vi "0037-0001_SHT31.vi"() -> ()   [LabVIEW 2014]
panel:
  out "x = y?":bool
  out "湿度":dbl format="%.2g"
  out "温度":dbl format="%.2g"
  in  "停止ボタン":bool
  # "℃"
  # "％RH"
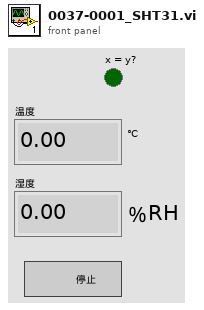
[diagram p1: front panel]
types:
  T1 = cluster{"bitRate":u32, "address":u8, "autoReadRespond":bool, "writeTimeout":u16, "readTimeout":u16, "sclLowTimeout":bool, "transferRetries":u16}
  T2 = typedef "CP2112_device.ctl" = i32
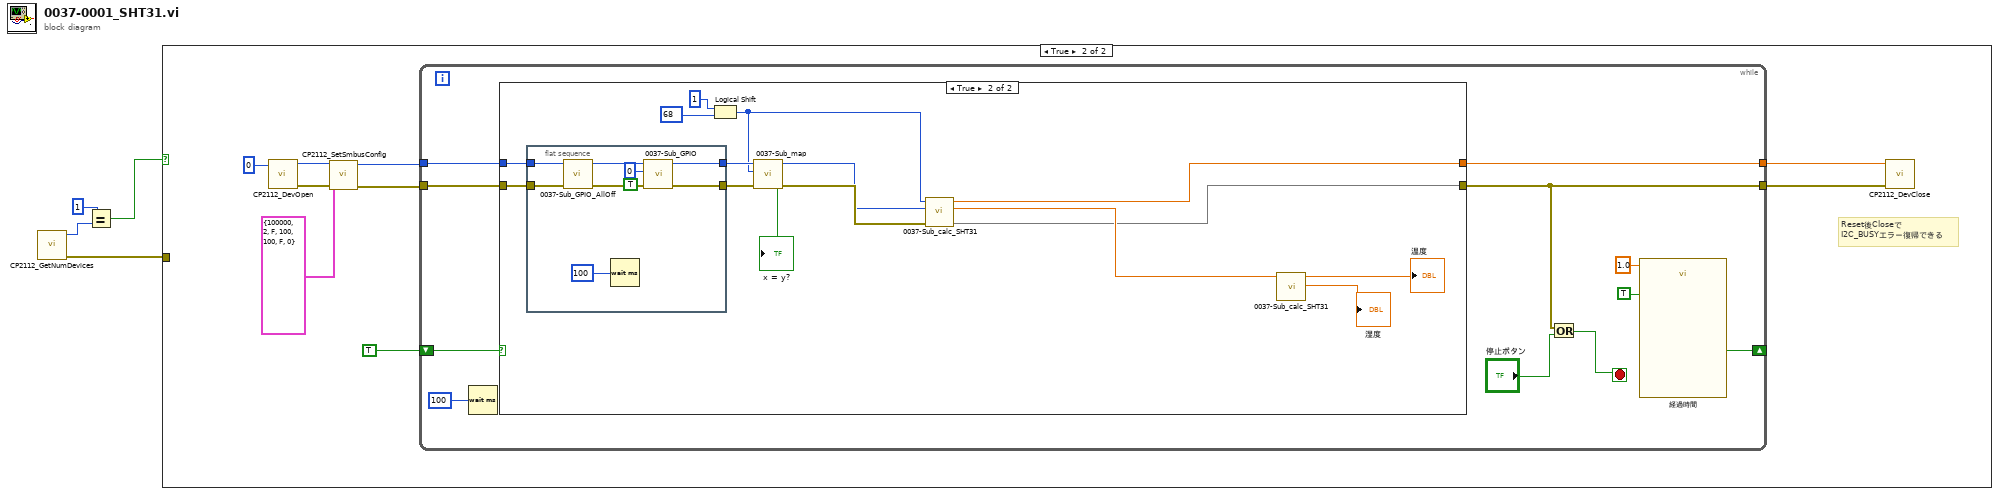
[diagram p0: block diagram]
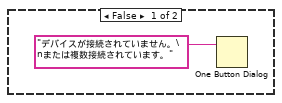
[diagram p2: hidden frame]
diagram:
  n1 = call <userlib>:"CP2112_GetNumDevices.vi"() -> ("error out"=w1:errorcluster, "numDevices"=w3:i32)  [unwired: 9 in, 1 out]
  n2 = Equal?(x=1, y=w3) -> (x = y?=w2:bool)
  n3 = case shown="TRUE" w2 {
    tunnel: w1 -> [_ _]
    frame False {
      n4 = One Button Dialog(message="デバイスが接続されていません。\nまたは複数接続されています。" ("メッセージ")) -> ()  [unwired: 1 in, 1 out]
    }
    frame True {
      # "Reset後Closeで\nI2C_BUSYエラー復帰できる"
      n5 = call <userlib>:"CP2112_DevOpen.vi"("deviceNum"=0) -> ("error out"=w9:errorcluster, "device"=w10:T2)  [unwired: 8 in, 1 out]
      n6 = call <userlib>:"CP2112_SetSmbusConfig.vi"("error in (no error)"=w9, "smbusInfo"=T1 {"bitRate"=100000, "address"=2, "autoReadRespond"=FALSE, "writeTimeout"=100, "readTimeout"=100, "sclLowTimeout"=FALSE, "transferRetries"=0}, "device"=w10) -> ("error out"=w11:errorcluster, "deviceOut"=w12:T2)  [unwired: 6 in, 1 out]
      n7 = while {
        tunnel: w11 -> [w25]
        tunnel: w12 -> [w24]
        tunnel: [w21] -> w7
        tunnel: [w20] -> w6
        shift-right: [w17] -> _
        shift-left: TRUE ("Auto Reset") -> [w18]
        stop <- w22 stop-if-true
        n8 = Wait (ms)(milliseconds to wait=u32 100 ("ミリ秒待機時間")) -> ()  [unwired: 1 out]
        n9 = case shown="TRUE" w18 {
          tunnel: w25 -> [w26 w33]
          tunnel: w24 -> [w27 w34]
          tunnel: [w26 w36] -> w21
          tunnel: [w27 w35] -> w20
          frame False {
          }
          frame True {
            n10 = flat-sequence {
              tunnel: w34 -> [w51]
              tunnel: w33 -> [w48]
              tunnel: [w49] -> w32
              tunnel: [w46] -> w31
              frame #0 {
                n11 = call "0037-Sub_GPIO_AllOff.vi"("エラー出力 2"=w48, "device"=w51) -> ("エラー出力"=w47:errorcluster, "deviceOut"=w50:T2)  [unwired: 8 in]
                n12 = Wait (ms)(milliseconds to wait=u32 100 ("ミリ秒待機時間")) -> ()  [unwired: 1 out]
                n13 = call "0037-Sub_GPIO.vi"("エラー出力 2"=w47, "ブール"=TRUE, "GPIO"=u8 0, "device"=w50) -> ("エラー出力"=w46:errorcluster, "deviceOut"=w49:T2)  [unwired: 6 in]
              }
            }
            n14 = Logical Shift(y=1, x=68) -> (x << y=w28:i32)
            n15 = call "0037-Sub_map.vi"("error out"=w31, "アドレス"=w28, "device"=w32) -> ("error out 2"=w39:errorcluster, "x = y?"=→"x = y?":bool, "device 2"=w38:T2)  [unwired: 5 in]
            n16 = call "0037-Sub_calc_SHT31.vi"(8:w39, 10:w38, "Data"=w28) -> (0:w36, "数値"=w42:dbl, "数値 2"=w35:dbl)  [unwired: 6 in]
            n17 = call "0037-Sub_calc_SHT31.vi"("Data"=w42) -> ("数値"=→"湿度":dbl, "数値 2"=→"温度":dbl)  [unwired: 9 in]
          }
        }
        n18 = Or(x=w21, y="停止ボタン") -> (x .or. y?=w22:bool)
        n19 = call "経過時間"("Time Target (s)"=1.0, "Auto Reset"=TRUE) -> ("Time has Elapsed"=w17:bool)  [unwired: 10 in, 7 out]
      }
      n20 = call <userlib>:"CP2112_DevClose.vi"("error in (no error)"=w7, "device"=w6) -> ()  [unwired: 9 in, 1 out]
    }
  }
